vi "file -- read-write segment file -- atomic.vi"(0 "sweep folder path":path, 1 "segment file action":T2, 2 "segment file kind":T1=enum."monitor, _m", 7 "temperatures IN":dbl[](array[numeric]), 9 "segment IN":dbl[][](array[numeric]), 11 "header IN":string[](array[string]), 12 "temperature":dbl, 14 "frequency":dbl) -> (4 "sweep folder path out":path, 8 "temperatures":dbl[](array[numeric]), 10 "segment":dbl[][](array[numeric]), 15 "header":string[](array[string]))   [LabVIEW 2014]
uses:
  segment file -- action.ctl
  segment file kind.ctl
  <vilib>/Utility/libraryn.llb/Check if File or Folder Exists.vi
panel:
  out "timestamp string array":string[](array[string])
  out "time (min)":dbl[](array[numeric])
  in  "segment":i32=10000
  in  "freq":i32=10000
  in  "significant digits":i32=10000
  out "number":i32=9
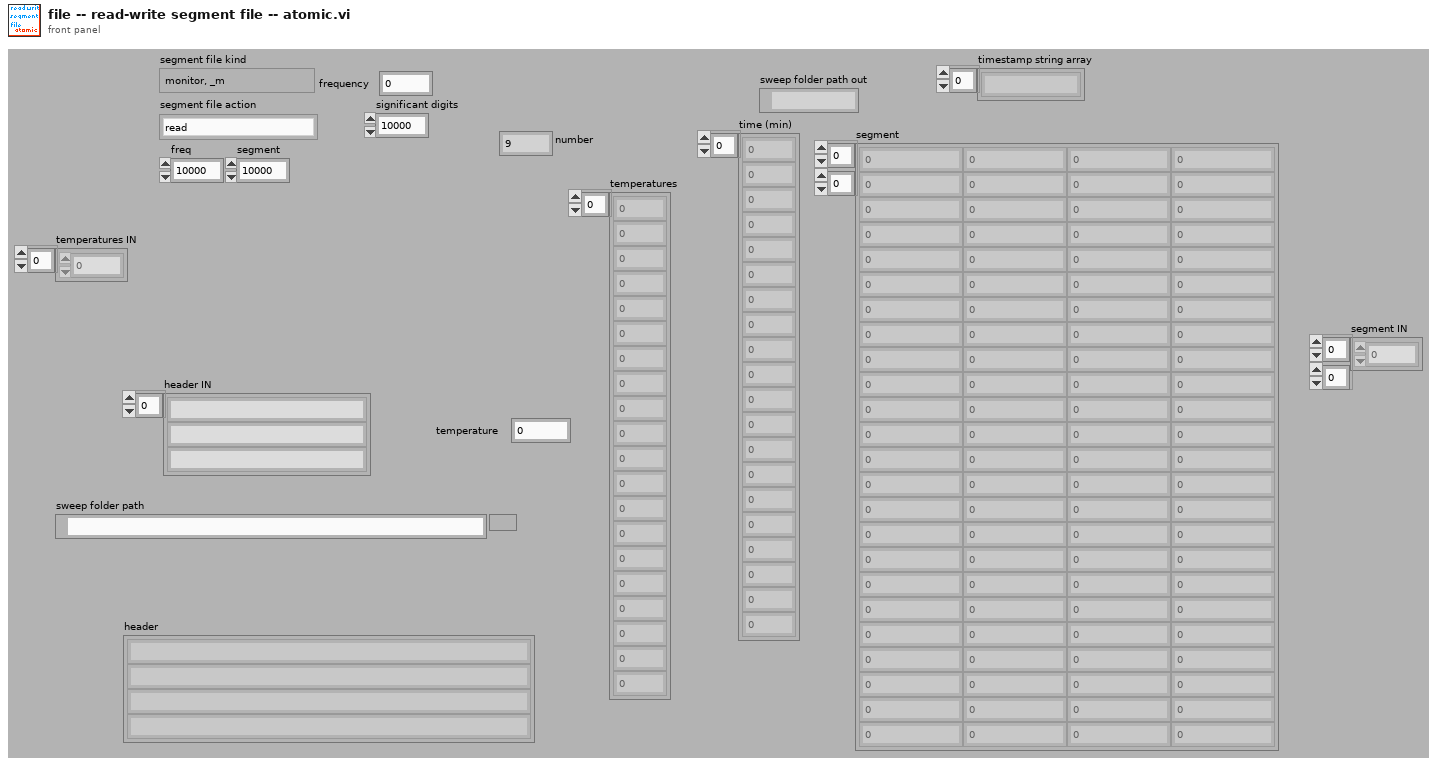
[diagram p1: front panel]
types:
  T1 = typedef "segment file kind.ctl" = enum16{"segments, _a", "monitor, _m", "other"}
  T2 = typedef "segment file -- action.ctl" = enum16{"read", "interpolate", "append col", "write", "write PID col", "append PID col"}
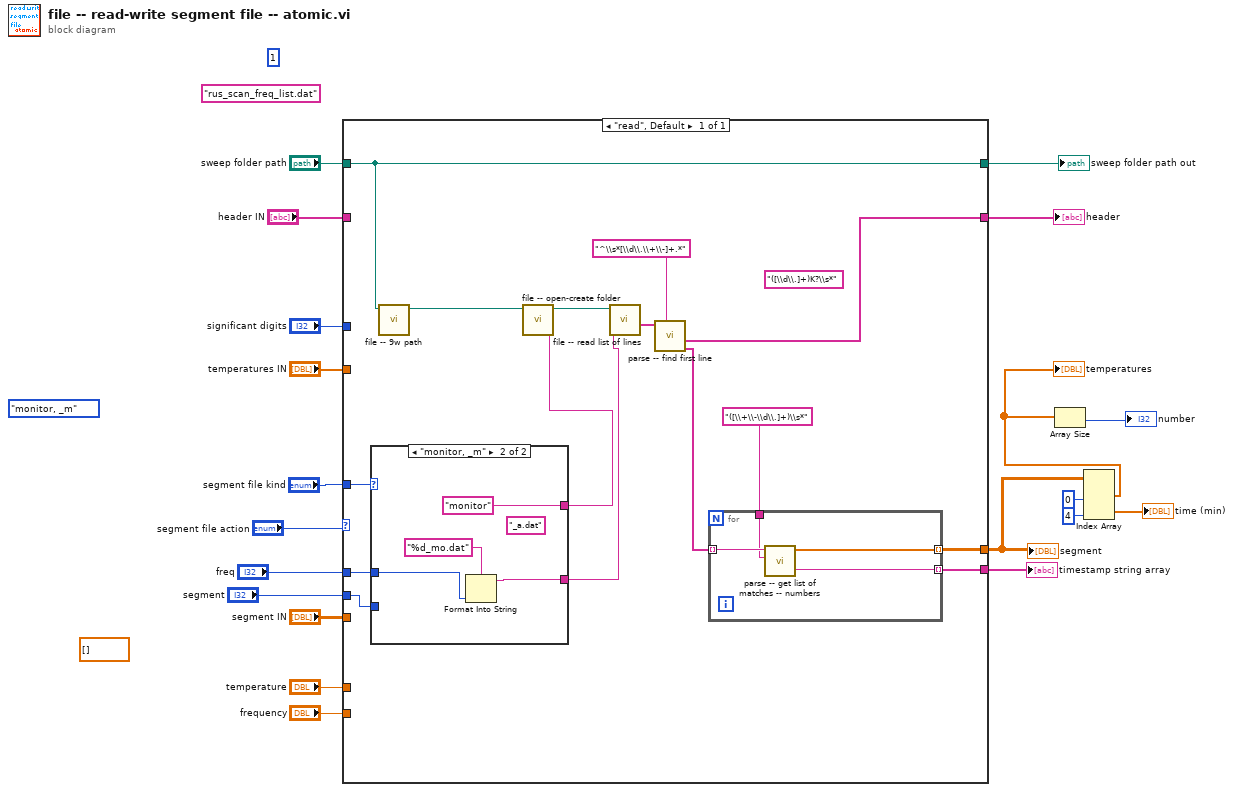
[diagram p0: block diagram]
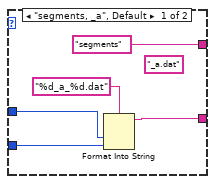
[diagram p2: hidden frame]
diagram:
  (unwired) segment_file_kind."monitor, _m" ("segment file kind")
  (unwired) dbl[] []
  (unwired) 1
  (unwired) "rus_scan_freq_list.dat" ("delimiter (\\t)")
  n1 = case shown="\"read\", Default" "segment file action" {
    tunnel: [w35] -> w6
    tunnel: "temperature" -> [_]
    tunnel: "sweep folder path" -> [w34]
    tunnel: "temperatures IN" -> [_]
    tunnel: "segment IN" -> [_]
    tunnel: "frequency" -> [_]
    tunnel: [w34] -> w16
    tunnel: [w32] -> w13
    tunnel: "header IN" -> [_]
    tunnel: "significant digits" -> [_]
    tunnel: "segment file kind" -> [w29]
    tunnel: "freq" -> [w26]
    tunnel: "segment" -> [w25]
    tunnel: [w21] -> w1
    frame "read", Default {
      (unwired) "([\\d\\.]+)K?\\s*" ("regexp")
      n2 = case shown="\"monitor, _m\"" w29 {
        tunnel: ["segments" ("name or relative path") "monitor" ("name or relative path")] -> w28
        tunnel: w26 -> [w38 w42]
        tunnel: w25 -> [w37 _]
        tunnel: [w36 w41] -> w24
        frame "segments, _a", Default {
          (unwired) "_a.dat" ("name or relative path")
          n3 = Format Into String(format string="%d_a_%d.dat", w38, w37) -> (resulting string=w36:string)  [unwired: 2 in, 1 out]
        }
        frame "monitor, _m" {
          (unwired) "_a.dat" ("name or relative path")
          n4 = Format Into String(format string="%d_mo.dat", w42) -> (resulting string=w41:string)  [unwired: 2 in, 1 out]
        }
      }
      n5 = call "file -- 9w path.vi"("sweep folder"=w34) -> ("9w path"=w30:path)  [unwired: 10 in]
      n6 = call "file -- open-create folder.vi"("folder name"=w28, "base path"=w30) -> ("folder path out"=w27:path)  [unwired: 9 in]
      n7 = call "file -- read list of lines.vi"("file name"=w24, "folder path"=w27) -> ("text lines"=w31:string[])  [unwired: 9 in]
      n8 = call "parse -- find first line.vi"("regexp"="^\\s*[\\d\\.\\+\\-]+.*", "string array"=w31) -> ("line and after"=w23:string[], "before"=w32:string[])  [unwired: 5 in, 3 out]
      n9 = for {
        tunnel: [w48] -> w35 mode=indexing
        tunnel: w23 -> [w47] mode=indexing
        tunnel: "([\\+\\-\\d\\.]+)\\s*" ("regexp") -> [w46]
        tunnel: [w45] -> w21 mode=indexing
        n10 = call "parse -- get list of matches -- numbers.vi"("regexp"=w46, "string"=w47) -> ("after match"=w45:string, "Array of numbers"=w48:dbl[])  [unwired: 6 in, 2 out]
      }
    }
  }
  "segment" <- w6
  "sweep folder path out" <- w16
  "header" <- w13
  "timestamp string array" <- w1
  n11 = Index Array(array=w6, index (col) #1=0 ("disabled index (col)"), index (col) #2=4 ("index (col)")) -> (element #1=w4:dbl[], element #2=→"time (min)":dbl[])  [unwired: 2 in]
  "temperatures" <- w4
  n12 = Array Size(array=w4) -> (size(s)=→"number":i32)
